vi "Update_FFID_Bkgnd_info.vi"(1 "First Bknd since calib":bool, 2 "c^2 (ppm^2)":dbl[](array[numeric]), 3 "Specific Bkgnd Meas?":bool, 4 "C (ppm)":dbl[](array[numeric])) -> ()   [LabVIEW 2017]
uses:
  Globals/Meas_global.vi
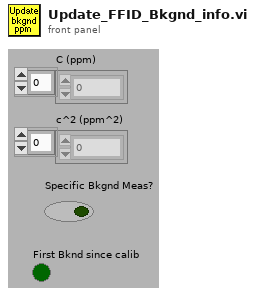
[diagram p1: front panel]
types:
  T1 = typedef "Analysis_info_cluster.ctl" = cluster{"Colour":u32, "Inst type":T2, "Inst name":string, "Symbol":string, "Code name":string, "Extra Info":string, "Inst Array":T3, "Extra Titles":string[], "Extra Values":string[], "U":dbl, "u^2":dbl, "u^3":dbl, "u^4":dbl, "Skew_u":dbl, "Kurt_u":dbl, "Sd Error in Mean":dbl, "% u'/U":dbl, "X":dbl, "Y":dbl, "Z":dbl, "Timescale integral Estimate":dbl, "Sd Error in Variance":dbl, "Calib File":path, "Calib Constants":dbl[], "Output Position":bool, "Full Stats":bool, "Av Sampling Rate":dbl, "Av No of Samples":dbl, "Total Meas Time (s)":dbl, "ADAM Ch Name":string, "Max value":dbl, "Min value":dbl}
  T2 = typedef "Inst_type.ctl" = enum16{"Propeller anemometer", "Raw voltage", "Pressure Transducer", "Pitot-static tube", "Preston tube", "Hot wire", "Cross wire 1", "Cross wire 2", "Generic Linear", "Generic Polynomial", "Generic BackPoly", "Fast FID", "Thermocouple", "Cold wire", "Pulsed Wire", "LDA Vel", "LDA Tran time", "LDA Arr time", "Microphone"}
  T3 = typedef "Instrument_Array.ctl" = enum16{"PWA", "LDA", "Analogue"}
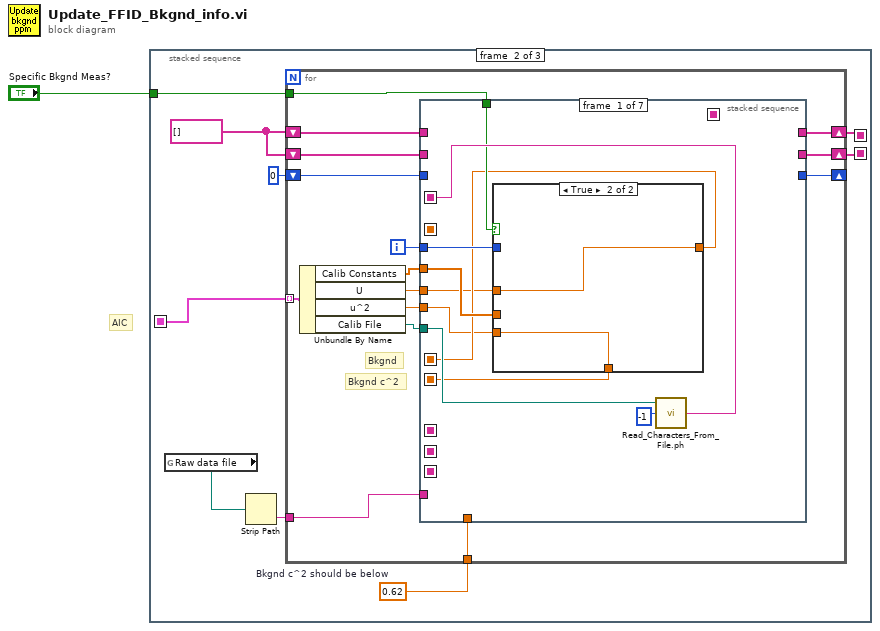
[diagram p0: block diagram]
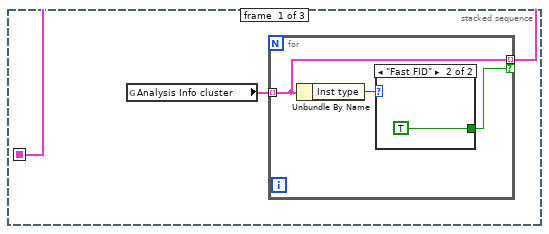
[diagram p2: hidden frame]
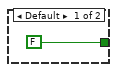
[diagram p3: hidden frame]
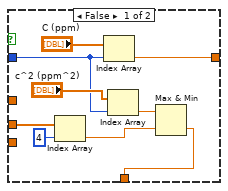
[diagram p4: hidden frame]
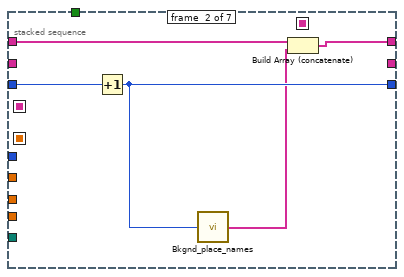
[diagram p5: hidden frame]
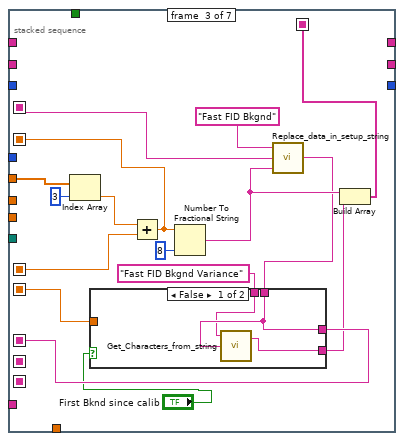
[diagram p6: hidden frame]
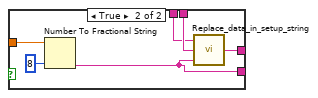
[diagram p7: hidden frame]
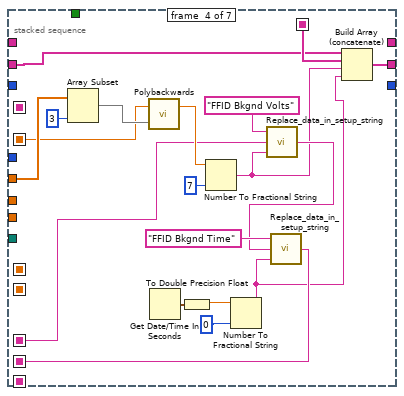
[diagram p8: hidden frame]
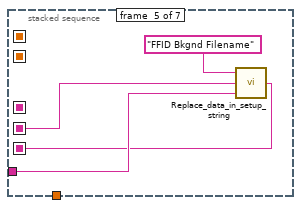
[diagram p9: hidden frame]
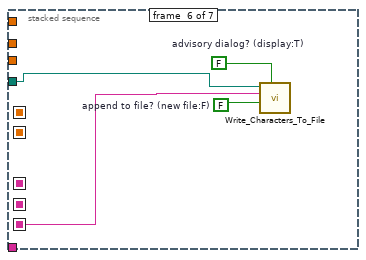
[diagram p10: hidden frame]
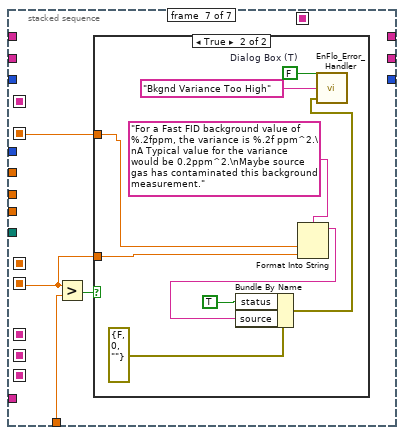
[diagram p11: hidden frame]
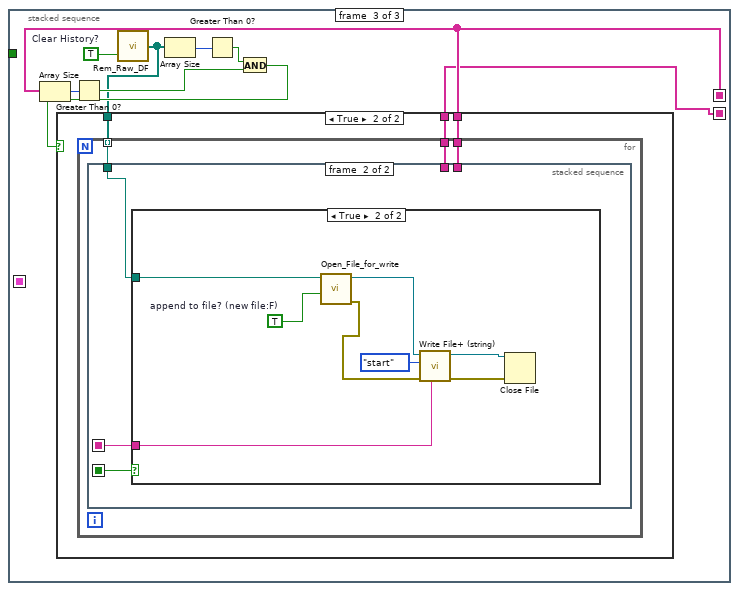
[diagram p13: hidden frame]
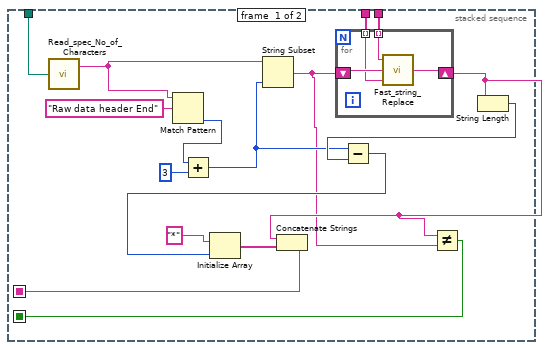
[diagram p15: hidden frame]
diagram:
  # "AIC"
  n1 = stacked-sequence {
    seq-local: [_ w13 _] -> [_ _ w126]
    seq-local: [_ w12 _] -> [_ _ w125]
    seq-local: [w2 _ _] -> [_ w10 _]
    tunnel: "Specific Bkgnd Meas?" -> [_ w9 _]
    frame #0 {
      n2 = global read "Meas_global.vi" "Analysis Info cluster"() -> (w3:T1[])
      n3 = for {
        tunnel: w3 -> [w6] mode=indexing
        tunnel: [w6] -> w2 mode=indexing if=w4
        n4 = Unbundle By Name(w6) -> ("Inst type"=w5:T2)
        n5 = case shown="\"Fast FID\"" w5 {
          tunnel: [FALSE TRUE] -> w4
          frame Default {
          }
          frame "Fast FID" {
          }
        }
      }
    }
    frame #1 {
      w11 = 0.62  # Bkgnd c^2 should be below
      w14 = string[] []
      n6 = global read "Meas_global.vi" "Raw data file"() -> (w17:path)
      n7 = Strip Path(path=w17) -> (name=w16:string)  [unwired: 1 out]
      n8 = for {
        tunnel: w16 -> [w32]
        shift-right: [w30] -> _
        shift-left: 0 -> [w31]
        shift-right: [w26] -> w12
        shift-left: w14 -> [w27]
        shift-right: [w28] -> w13
        shift-left: w14 -> [w29]
        tunnel: w11 -> [w25]
        tunnel: w10 -> [w22] mode=indexing
        tunnel: w9 -> [w24]
        i -> [w23]
        # "Bkgnd c^2"
        # "Bkgnd"
        n9 = Unbundle By Name(w22) -> ("Calib Constants"=w21:dbl[], "U"=w20:dbl, "u^2"=w18:dbl, "Calib File"=w19:path)
        n10 = stacked-sequence {
          seq-local: [w41 _ _ _ _ _ _] -> [_ _ w69 _ _ _ _]
          seq-local: [_ _ w68 _ _ _ _] -> [_ _ _ w91 _ _ _]
          seq-local: [_ _ w67 _ _ _ _] -> [_ _ _ w99 _ _ w114]
          seq-local: [_ _ _ w89 _ _ _] -> [_ _ _ _ w103 _ _]
          seq-local: [_ _ _ _ w104 _ _] -> [_ _ _ _ _ w108 _]
          seq-local: [_ _ w63 _ _ _ _] -> [_ _ _ w88 _ _ _]
          seq-local: [w38 _ _ _ _ _ _] -> [_ _ w62 _ _ _ w113]
          seq-local: [w35 _ _ _ _ _ _] -> [_ _ w61 _ _ _ _]
          tunnel: w21 -> [w37 _ w74 w102 _ _ _]
          tunnel: w19 -> [w40 _ _ _ _ w107 _]
          tunnel: w32 -> [_ _ _ _ w105 _ _]
          tunnel: w31 -> [_ w58 _ _ _ _ _]
          tunnel: [_ w57 _ _ _ _ _] -> w30
          tunnel: w29 -> [_ w55 _ _ _ _ _]
          tunnel: [_ w54 _ _ _ _ _] -> w28
          tunnel: w27 -> [_ _ _ w85 _ _ _]
          tunnel: [_ _ _ w84 _ _ _] -> w26
          tunnel: w25 -> [_ _ _ _ _ _ w111]
          tunnel: w24 -> [w39 _ _ _ _ _ _]
          tunnel: w23 -> [w36 _ _ _ _ _ _]
          tunnel: w20 -> [w34 _ _ _ _ _ _]
          tunnel: w18 -> [w33 _ _ _ _ _ _]
          frame #0 {
            n11 = case shown="True" w39 {
              tunnel: [w43 w52] -> w38
              tunnel: w37 -> [w51 _]
              tunnel: w36 -> [w46 _]
              tunnel: [w48 w53] -> w35
              tunnel: w34 -> [_ w53]
              tunnel: w33 -> [_ w52]
              frame False {
                n12 = Index Array(array=w51, index=4) -> (element=w44:dbl)
                n13 = Index Array(array="C (ppm)", index=w46) -> (element=w48:dbl)
                n14 = Index Array(array="c^2 (ppm^2)", index=w46) -> (element=w45:dbl)
                n15 = Max & Min(x=w45, y=w44) -> (min(x,y)=w43:dbl)  [unwired: 1 out]
              }
              frame True {
              }
            }
            n16 = call "Read_Characters_From_File.ph.vi"("file path (dialog if empty)"=w40, "number of characters (all:-1)"=-1) -> ("character string"=w41:string)  [unwired: 7 out]
          }
          frame #1 {
            n17 = Increment(x=w58) -> (x+1=w57:i32)
            n18 = call "Bkgnd_place_names.vi"("Numeric"=w57) -> ("Array"=w56:string[])
            n19 = Build Array (concatenate)(w55, w56) -> (w54:string[])
          }
          frame #2 {
            n20 = Index Array(array=w74, index=3 ("Index")) -> (element=w72:dbl)
            n21 = Add(x=w72, y=w61) -> (x+y=w67:dbl)
            n22 = Number To Fractional String(number=w67, precision (6)=i16 8) -> (F-format string=w66:string)  [unwired: 2 out]
            n23 = call "Replace_data_in_setup_string.vi"("New data string"=w66, "Input string"=w69, "Variable name"="Fast FID Bkgnd") -> ("Appended string"=w65:string)
            n24 = case shown="False" "First Bknd since calib" {
              tunnel: [w77 w83] -> w68
              tunnel: w65 -> [w77 w81]
              tunnel: [w75 w80] -> w64
              tunnel: w62 -> [_ w79]
              tunnel: "Fast FID Bkgnd Variance" -> [w76 w78]
              frame False {
                n25 = call "Get_Characters_from_string.vi"("Input string"=w77, "Variable name"=w76) -> ("Value"=w75:string)  [unwired: 1 in, 1 out]
              }
              frame True {
                n26 = Number To Fractional String(number=w79, precision (6)=i16 8) -> (F-format string=w80:string)  [unwired: 2 out]
                n27 = call "Replace_data_in_setup_string.vi"("New data string"=w80, "Input string"=w81, "Variable name"=w78) -> ("Appended string"=w83:string)
              }
            }
            n28 = Build Array(w66, w64) -> (w63:string[])
          }
          frame #3 {
            n29 = Array Subset(array=w102, length=3 ("index")) -> (w100:dbl[])  [unwired: 1 in]
            n30 = call "Polybackwards.vi"("Coefficients"=w100, "Y input"=w99) -> ("X output"=w98:dbl)  [unwired: 1 out]
            n31 = Get Date/Time In Seconds() -> (seconds since 1Jan1904=w95:timestamp)
            n32 = To Double Precision Float(number=w95) -> (double precision float=w93:dbl)
            n33 = Number To Fractional String(number=w98, precision (6)=i16 7) -> (F-format string=w87:string)  [unwired: 2 out]
            n34 = Number To Fractional String(number=w93, precision (6)=i16 0) -> (F-format string=w86:string)  [unwired: 2 out]
            n35 = call "Replace_data_in_setup_string.vi"("New data string"=w87, "Input string"=w91, "Variable name"="FFID Bkgnd Volts") -> ("Appended string"=w90:string)
            n36 = call "Replace_data_in_setup_string.vi"("New data string"=w86, "Input string"=w90, "Variable name"="FFID Bkgnd Time") -> ("Appended string"=w89:string)
            n37 = Build Array (concatenate)(w85, w88, w87, w86) -> (w84:string[])
          }
          frame #4 {
            n38 = call "Replace_data_in_setup_string.vi"("New data string"=w105, "Input string"=w103, "Variable name"="FFID Bkgnd Filename") -> ("Appended string"=w104:string)
          }
          frame #5 {
            w109 = FALSE  # advisory dialog? (display:T)
            w110 = FALSE  # append to file? (new file:F)
            n39 = call "Write_Characters_To_File.vi"("file path (dialog if empty)"=w107, "advisory dialog? (display:T)"=w109, "character string"=w108, "append to file? (new file:F)"=w110) -> ()  [unwired: 1 in, 4 out]
          }
          frame #6 {
            n40 = Greater?(x=w113, y=w111) -> (0:w112:bool)
            n41 = case shown="True" w112 {
              tunnel: w113 -> [_ w120]
              tunnel: w114 -> [_ w119]
              frame False {
              }
              frame True {
                w115 = FALSE  # Dialog Box (T)
                n42 = Format Into String(format string="For a Fast FID background value of %.2fppm, the variance is %.2f ppm^2.\nA Typical value for the variance would be 0.2ppm^2.\nMaybe source gas has contaminated this background measurement.", w119, w120) -> (resulting string=w117:string)  [unwired: 2 in, 1 out]
                n43 = Bundle By Name(cluster=errorcluster {"status"=FALSE, "code"=0, "source"=""} ("error in (no error)"), "status"=TRUE, "source"=w117) -> (w116:errorcluster)
                n44 = call "EnFlo_Error_Handler.vi"("error in (no error)"=w116, "Error Type"="Bkgnd Variance Too High", "Dialog Box (T)"=w115) -> ()  [unwired: 3 out]
              }
            }
          }
        }
      }
    }
    frame #2 {
      w124 = TRUE  # Clear History?
      n45 = Array Size(array=w126) -> (size(s)=w131:i32)
      n46 = Greater Than 0?(x=w131) -> (x > 0?=w129:bool)
      n47 = call "Rem_Raw_DF.vi"("Clear History?"=w124) -> ("List of Filenames"=w127:path[])  [unwired: 1 in]
      n48 = Array Size(array=w127) -> (size(s)=w132:i32)
      n49 = Greater Than 0?(x=w132) -> (x > 0?=w130:bool)
      n50 = And(x=w130, y=w129) -> (x .and. y?=w128:bool)
      n51 = case shown="True" w128 {
        tunnel: w127 -> [_ w135]
        tunnel: w126 -> [_ w134]
        tunnel: w125 -> [_ w133]
        frame False {
        }
        frame True {
          n52 = for {
            tunnel: w135 -> [w136] mode=indexing
            tunnel: w134 -> [w138]
            tunnel: w133 -> [w137]
            n53 = stacked-sequence {
              seq-local: [w142 _] -> [_ w160]
              seq-local: [w140 _] -> [_ w159]
              tunnel: w138 -> [w150 _]
              tunnel: w137 -> [w149 _]
              tunnel: w136 -> [w143 w161]
              frame #0 {
                n54 = call "Read_spec_No_of_Characters.vi"("Filename"=w143) -> ("character string"=w151:string)  [unwired: 1 out]
                n55 = Match Pattern(string=w151, regular expression="Raw data header End") -> (offset past match=w153:i32)  [unwired: 4 out]
                n56 = Add(x=w153, y=3) -> (x+y=w147:i32)
                n57 = String Subset(string=w151, length (rest)=w147) -> (substring=w139:string)  [unwired: 1 out]
                n58 = for {
                  shift-right: [w157] -> w141
                  shift-left: w139 -> [w158]
                  tunnel: w150 -> [w156] mode=indexing
                  tunnel: w149 -> [w155] mode=indexing
                  n59 = call "Fast_string_Replace.vi"("Replace match with:"=w155, "Input String"=w158, "regular expression"=w156) -> ("Output String"=w157:string)  [unwired: 2 out]
                }
                n60 = Not Equal?(x=w141, y=w139) -> (x != y?=w140:bool)
                n61 = String Length(string=w141) -> (length=w148:i32)
                n62 = Subtract(x=w147, y=w148) -> (x-y=w145:i32)
                n63 = Initialize Array("*", w145) -> (w144:string[])
                n64 = Concatenate Strings(w141, w144) -> (w142:string)
              }
              frame #1 {
                n65 = case shown="True" w159 {
                  tunnel: w161 -> [_ w169]
                  tunnel: w160 -> [_ w162]
                  frame False {
                  }
                  frame True {
                    w168 = TRUE  # append to file? (new file:F)
                    n66 = call "Open_File_for_write.vi"("append to file? (new file:F)"=w168, "file path"=w169) -> ("error out"=w165:errorcluster, "refnum"=w166:refnum<file>)  [unwired: 1 in, 7 out]
                    n67 = call <vilib>:"Write File+ (string).vi"("string"=w162, "error in (no error)"=w165, "pos mode (rel. to end:1)"=enum16{"start", "end", "current"}."start", "refnum"=w166) -> ("error out"=w163:errorcluster, "dup refnum"=w164:refnum<file>)  [unwired: 1 in, 3 out]
                    n68 = Close File(refnum=w164, error in=w163) -> ()  [unwired: 2 out]
                  }
                }
              }
            }
          }
        }
      }
    }
  }
